vi "Get value string.vi"(8 "error in (no error)":errorcluster, 10 "Replace FKs? (F)":bool, 11 "Column in":refnum<class "Composed Column.lvclass">) -> (0 "error out":errorcluster, 1 "Default?":bool, 2 "Value":string, 3 "Column out":refnum<class "Composed Column.lvclass">)   [LabVIEW 2020, in "Composed Columns.lvlib" / "Composed Column.lvclass"]
uses:
  Composed Column.lvclass
  Composed Column.lvclass/Composed Column.ctl
  Value Type/Value Type.lvclass
  Composed Columns/Value Source Interface Class/Value Source.lvclass
  Basic Columns/Column Configuration/Basic Column Configuration Class/Column Configuration.lvclass
  Database Libraries/Database Interfaces/Database Interface Class/Database Interface.lvclass
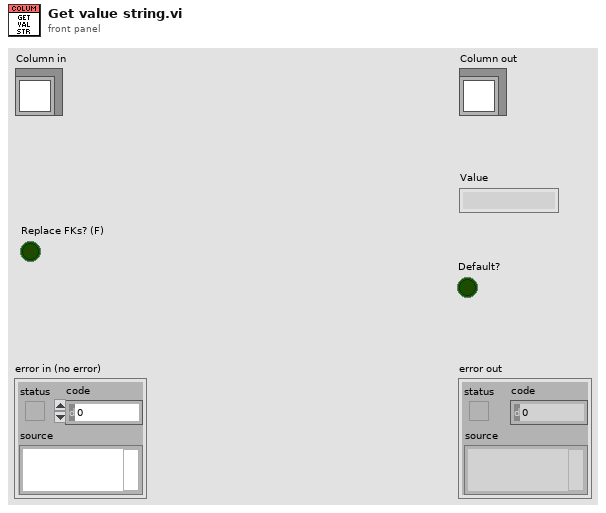
[diagram p1: front panel]
types:
  T1 = typedef "Column Interfaces.lvlib/FK Info.ctl" = cluster{"PK Table":string, "PK Column":string, "PK Display Column":string}
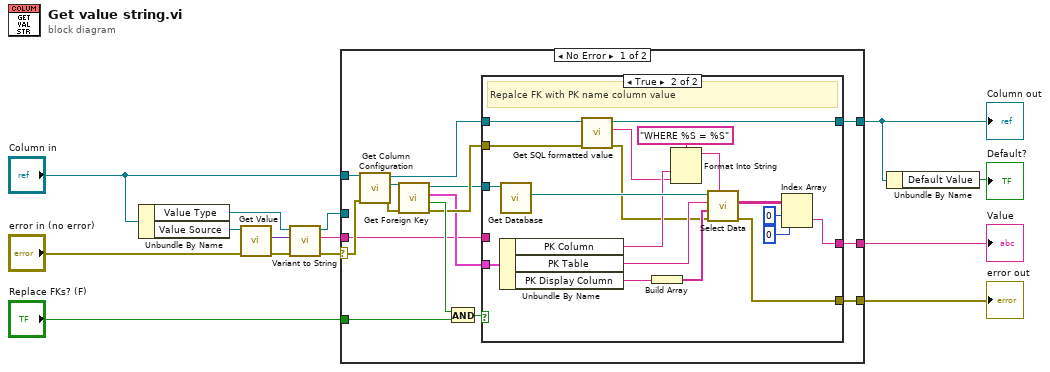
[diagram p0: block diagram]
diagram:
  n1 = Unbundle By Name("Column in") -> ("Value Type"=w14:refnum<class "Value Type.lvclass">, "Value Source"=w13:refnum<class "Value Source.lvclass">)
  n2 = call-dynamic "Get Value.vi"("error in (no error)"="error in (no error)", "Value Source in"=w13) -> ("error out"=w10:errorcluster, "Value"=w12:variant)  [unwired: 7 in, 1 out]
  n3 = call-dynamic "Variant to String.vi"("error in (no error)"=w10, "Variant"=w12, "Value Type in"=w14) -> ("error out"=w8:errorcluster, "String"=w4:string, "Value Type out"=w7:refnum<class "Value Type.lvclass">)  [unwired: 6 in]
  n4 = case shown="No Error" w8 {
    selector: w8 -> [w24 w53]
    tunnel: [w18 w54] -> w2
    tunnel: "Column in" -> [w29 w54]
    tunnel: w7 -> [_ _]
    tunnel: [w16 w53] -> w6
    tunnel: "Replace FKs? (F)" -> [w25 _]
    tunnel: w4 -> [w15 w52]
    tunnel: [w17 w52] -> w3
    frame No Error {
      n5 = call-dynamic "Get Column Configuration.vi"("error in (no error)"=w24, "Composed Column in"=w29) -> ("error out"=w23:errorcluster, "Column Configuration"=w28:refnum<class "Column Configuration.lvclass">, "Composed Column out"=w19:refnum<class "Composed Column.lvclass">)  [unwired: 7 in]
      n6 = call-dynamic "Get Foreign Key.vi"("error in (no error)"=w23, "Basic Column Configuration in"=w28) -> ("error out"=w22:errorcluster, "Is a FK?"=w26:bool, "FK Info"=w21:T1, "Basic Column Configuration out"=w20:refnum<class "Column Configuration.lvclass">)  [unwired: 6 in]
      n7 = And(x=w26, y=w25) -> (x .and. y?=w27:bool)
      n8 = case shown="True" w27 {
        tunnel: w22 -> [w31 w35]
        tunnel: w21 -> [_ w49]
        tunnel: w20 -> [_ w51]
        tunnel: w19 -> [w32 w43]
        tunnel: [w32 w41] -> w18
        tunnel: [w30 w36] -> w17
        tunnel: [w31 w33] -> w16
        tunnel: w15 -> [w30 _]
        frame False {
        }
        frame True {
          # "Repalce FK with PK name column value"
          n9 = Unbundle By Name(w49) -> ("PK Column"=w45:string, "PK Table"=w46:string, "PK Display Column"=w48:string)
          n10 = call-dynamic "Get Database.vi"("Basic Column Configuration in"=w51) -> ("Database"=w50:refnum<class "Database Interface.lvclass">)  [unwired: 8 in, 2 out]
          n11 = call-dynamic "Get SQL formatted value.vi"("error in (no error)"=w35, "Column in"=w43) -> ("error out"=w34:errorcluster, "Formatted Value"=w42:string, "Column out"=w41:refnum<class "Composed Column.lvclass">)  [unwired: 6 in, 1 out]
          n12 = Build Array(w48) -> (w47:string[])
          n13 = Format Into String(format string="WHERE %S = %S", w45, w42) -> (resulting string=w40:string)  [unwired: 2 in, 1 out]
          n14 = call-dynamic "Select Data.vi"("WHERE Statement"=w40, "error in (no error)"=w34, "Columns"=w47, "Table"=w46, "Database Interface in"=w50) -> ("error out"=w33:errorcluster, "Data"=w39:string[][])  [unwired: 4 in, 1 out]
          n15 = Index Array(array=w39, index (row)=0, index (col)=0 ("disabled index (col)")) -> (element=w36:string)
        }
      }
    }
    frame Error {
    }
  }
  "error out" <- w6
  "Column out" <- w2
  "Value" <- w3
  n16 = Unbundle By Name(w2) -> ("Default Value"=→"Default?":bool)
